vi "AlliGator Save Simulation Outputs to ASCII.vi"(8 "Error In":errorcluster, 9 "Fit Settings":T11 {"Decay Fit Options"."Confidence Level" min=0.0 max=100.0; "Decay Fit Options"."Offset Resolution" min=0.0; "Decay Fit Options"."Period" min=0.0; "Decay Fit Options"."Min Decay Percentile" min=0.0 max=1.0; "Decay Fit Options"."Max Decay Percentile" min=0.0 max=100.0; "Fit Parameter Constraints"."Max Value" format="%#.3g"; "Fit Parameter Constraints"."Min Value" format="%#.3g"}, 10 "Simulation Parameters Array":T12[](array[typedef]), 11 "Fit Results":cluster{"Fit Results":T15[]}[](array[cluster])) -> (0 "Error Out":errorcluster, 1 "Message":string)   [LabVIEW 2021, in "AlliGator Fit Method Benchmark.lvlib"]
doc: "Saves simulation results."
uses:
  AlliGator Fit Method Benchmark.lvlib
  Fits/IRF(X)PSED/IRF(X)PSED Fit Results.ctl
  AlliGator Simulation Parameters.ctl
  AlliGator Decay Simulation Parameters.ctl
  AlliGator Fit Simulation Parameters.ctl
  Fits/Decay Convolution/Decay Model.ctl
  Fits/Residual Type.ctl
  Fits/Non-linear Fitting Method v2.ctl
  Fits/Fit Calculation Method.ctl
  Fits/Non-linear Fitting Algorithm.ctl
  Decay Analysis/Decay Fit/AlliGator Decay Fit Parameter Constraints 2.ctl
  Fits/IRF(X)PSED/Decay Fit Parameters In List.ctl
  Fits/IRF(X)PSED/MLE Baseline Offset Type.ctl
  Files/Files.lvlib
  Strings/Strings.lvlib
  Fits/Fits.lvlib
  Decay Analysis/Decay Fit/AlliGator Decay Fit.lvlib
  Fits/IRF(X)PSED/Fit Weights Type v2.ctl
  Fits/IRF(X)PSED/Decay Fit Options v4.ctl
panel:
  in  "file (use dialog)":path
  # "see the AlliGator License on the block diagram (Ctrl+E or Window:Show Block Diagram)"
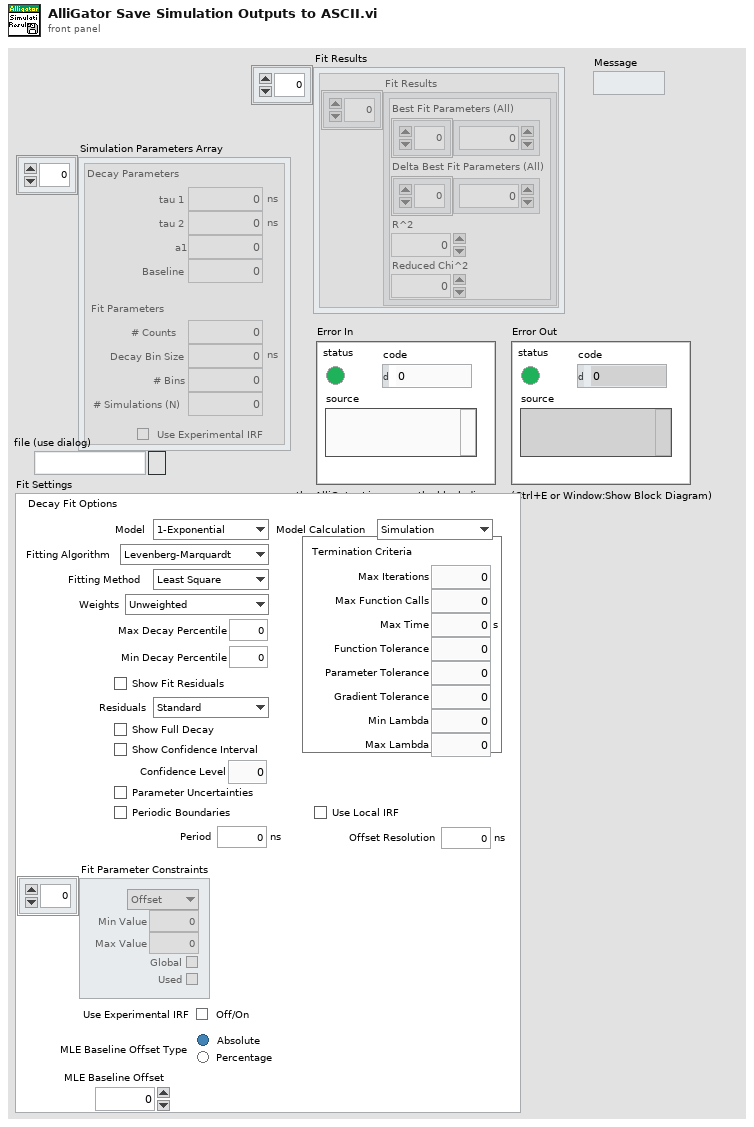
[diagram p1: front panel]
types:
  T1 = typedef "Fits.lvlib/Decay Fit Options v4.ctl" = cluster{"Show Fit Residuals":bool, "Fit Model":T2, "Residual Type":T3, "Max Decay Percentile":dbl, "Min Decay Percentile":dbl, "Show Full Decay":bool, "Weights":T4, "Fitting Method":T5, "Compute Parameter Uncertainties":bool, "Periodic Boundaries":bool, "Model Calculation":T6, "Period":dbl[unit], "Termination Criteria":cluster{"Max Iterations":i32, "Max Function Calls":i32, "Max Time":dbl[unit], "Function Tolerance":dbl, "Parameter Tolerance":dbl, "Gradient Tolerance":dbl, "Min Lambda":dbl, "Max Lambda":dbl, "Initial Tick Count":u32}, "Offset Resolution":dbl[unit], "Use Local IRF":bool, "Fitting Algorithm":T7, "Show Confidence Interval ":bool, "Confidence Level":dbl}
  T2 = typedef "Fits.lvlib/Decay Model.ctl" = enum16{"1-Exponential", "2-Exponentials"}
  T3 = typedef "Fits.lvlib/Residual Type.ctl" = enum16{"Standard", "Normalized", "Reduced"}
  T4 = typedef "Fits.lvlib/Fit Weights Type v2.ctl" = enum16{"Unweighted", "1/Variance (Neyman)", "1/Variance (Pearson)", "Best of All"}
  T5 = typedef "Fits.lvlib/Non-linear Fitting Method v2.ctl" = enum16{"Least Square", "Least Absolute Residual", "Bisquare", "MLE", "-", "Best of All"}
  T6 = typedef "Fits.lvlib/Fit Calculation Method.ctl" = enum16{"Simulation", "Convolution", "Integration"}
  T7 = typedef "Fits.lvlib/Non-linear Fitting Algorithm.ctl" = enum16{"Levenberg-Marquardt", "Trust-Region Dogleg"}
  T8 = typedef "AlliGator Decay Fit.lvlib/AlliGator Decay Fit Parameter Constraints 2.ctl" = cluster{"Fit Parameter":T9, "Min Value":dbl, "Max Value":dbl, "Global":bool, "Used":bool}
  T9 = typedef "Fits.lvlib/Decay Fit Parameters In List.ctl" = enum16{"Offset", "Baseline", "A_1", "tau_1", "A_2", "tau_2"}
  T10 = typedef "Fits.lvlib/MLE Baseline Offset Type.ctl" = enum32{"Absolute", "Percentage"}
  T11 = cluster{"Decay Fit Options":T1, "Fit Parameter Constraints":T8[], "Use Experimental IRF":bool, "MLE Baseline Offset Type":T10, "MLE Baseline Offset":dbl}
  T12 = typedef "AlliGator Fit Method Benchmark.lvlib/AlliGator Simulation Parameters.ctl" = cluster{"Decay Simulation Parameters":T13, "Fit Simulation Parameters":T14, "Use Experimental IRF":bool}
  T13 = typedef "AlliGator Fit Method Benchmark.lvlib/AlliGator Decay Simulation Parameters.ctl" = cluster{"tau 1":dbl[unit], "tau 2":dbl[unit], "a1":dbl, "Baseline":dbl}
  T14 = typedef "AlliGator Fit Method Benchmark.lvlib/AlliGator Fit Simulation Parameters.ctl" = cluster{"# Counts":i32, "# Simulations (N)":i32, "Decay Bin Size":dbl[unit], "# Bins":i32}
  T15 = typedef "Fits.lvlib/IRF(X)PSED Fit Results.ctl" = cluster{"Best Fit Parameters (All)":dbl[], "Delta Best Fit Parameters (All)":dbl[], "R^2":dbl, "Reduced Chi^2":dbl}
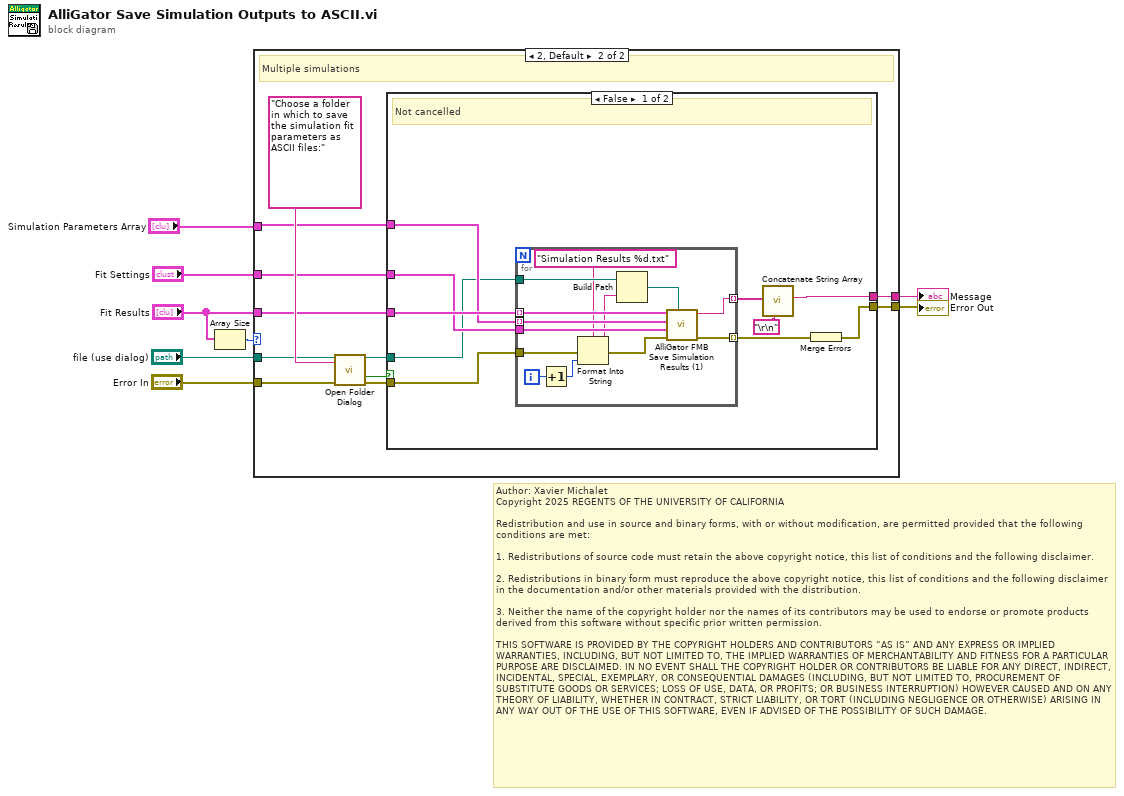
[diagram p0: block diagram]
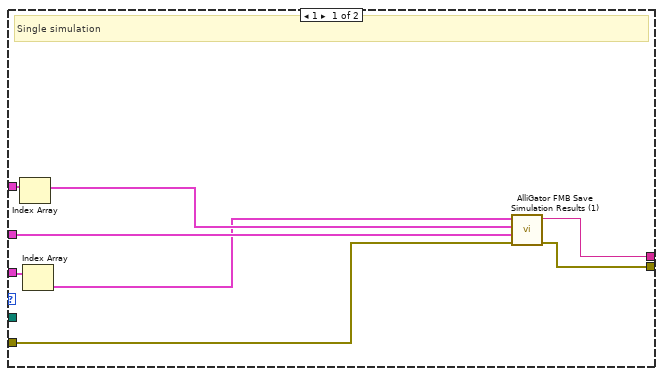
[diagram p2: hidden frame]
diagram:
  # "Author: Xavier Michalet\nCopyright 2025 REGENTS OF THE UNIVERSITY OF CALIFORNIA\n\nRedistribution and use in source and binary forms, with or without modification, are permitted provided that the following conditions are met:\n\n1. Redistributions of source code must retain the above copyright notice, this list of conditions and the following disclaimer.\n\n2. Redistributions in binary form must reproduce the above copyright notice, this list of conditions and the following disclaimer in the documentation and/or other materials provided with the distribution.\n\n3. Neither the name of the copyright holder nor the names of its contributors may be used to endorse or promote products derived from this software without specific prior written permission.\n\nTHIS SOFTWARE IS PROVIDED BY THE COPYRIGHT HOLDERS AND CONTRIBUTORS “AS IS” AND ANY EXPRESS OR IMPLIED WARRANTIES, INCLUDING, BUT NOT LIMITED TO, THE IMPLIED WARRANTIES OF MERCHANTABILITY AND FITNESS FOR A PARTICULAR PURPOSE ARE DISCLAIMED. IN NO EVENT SHALL THE COPYRIGHT HOLDER OR CONTRIBUTORS BE LIABLE FOR ANY DIRECT, INDIRECT, INCIDENTAL, SPECIAL, EXEMPLARY, OR CONSEQUENTIAL DAMAGES (INCLUDING, BUT NOT LIMITED TO, PROCUREMENT OF SUBSTITUTE GOODS OR SERVICES; LOSS OF USE, DATA, OR PROFITS; OR BUSINESS INTERRUPTION) HOWEVER CAUSED AND ON ANY THEORY OF LIABILITY, WHETHER IN CONTRACT, STRICT LIABILITY, OR TORT (INCLUDING NEGLIGENCE OR OTHERWISE) ARISING IN ANY WAY OUT OF THE USE OF THIS SOFTWARE, EVEN IF ADVISED OF THE POSSIBILITY OF SUCH DAMAGE."
  n1 = Array Size(array="Fit Results") -> (size(s)=w4:i32)
  n2 = case shown="2, Default" w4 {
    tunnel: "Error In" -> [w16 w26]
    tunnel: [w15 w17] -> w7
    tunnel: [w14 w19] -> w6
    tunnel: "Fit Results" -> [w10 w24]
    tunnel: "Simulation Parameters Array" -> [w12 w23]
    tunnel: "Fit Settings" -> [w13 w22]
    tunnel: "file (use dialog)" -> [_ w18]
    frame 1 {
      # "Single simulation"
      n3 = Index Array(array=w12) -> (element=w11:T12)  [unwired: 1 in]
      n4 = Index Array(array=w10) -> (element=w9:cluster{"Fit Results":T15[]})  [unwired: 1 in]
      n5 = call "AlliGator FMB Save Simulation Results (1).vi"("error in (no error)"=w16, "Fit Settings"=w13, "Simulation Parameters"=w11, "Fit Results"=w9) -> ("error out"=w15:errorcluster, "Message"=w14:string)  [unwired: 6 in]
    }
    frame 2, Default {
      # "Multiple simulations"
      n6 = call "Open Folder Dialog.vi"("start path"=w18, "prompt"="Choose a folder in which to save the simulation fit parameters as ASCII files:" ("prompt (Choose or enter file path)"), "error in"=w26) -> ("selected path"=w20:path, "cancelled"=w25:bool, "error out"=w21:errorcluster)  [unwired: 9 in, 1 out]
      n7 = case shown="False" w25 {
        tunnel: w24 -> [w37 _]
        tunnel: w23 -> [w36 _]
        tunnel: w22 -> [w35 _]
        tunnel: w21 -> [w34 w51]
        tunnel: w20 -> [w30 _]
        tunnel: [w32 _] -> w19
        tunnel: [w28 w51] -> w17
        frame False {
          # "Not cancelled"
          n8 = for {
            tunnel: w37 -> [w50] mode=indexing
            tunnel: w36 -> [w49] mode=indexing
            tunnel: w35 -> [w48]
            tunnel: w34 -> [w43]
            tunnel: [w47] -> w29 mode=indexing
            tunnel: [w46] -> w33 mode=indexing
            tunnel: w30 -> [w45]
            i -> [w42]
            n9 = Increment(x=w42) -> (x+1=w41:i32)
            n10 = Format Into String(format string="Simulation Results %d.txt", error in=w43, w41) -> (resulting string=w39:string, error out=w44:errorcluster)  [unwired: 1 in]
            n11 = Build Path(base path=w45, name or relative path=w39) -> (appended path=w38:path)
            n12 = call "AlliGator FMB Save Simulation Results (1).vi"("File Path (Dialog if empty)"=w38, "error in (no error)"=w44, "Fit Settings"=w48, "Simulation Parameters"=w49, "Fit Results"=w50) -> ("error out"=w47:errorcluster, "Message"=w46:string)  [unwired: 5 in]
          }
          n13 = call "Concatenate String Array.vi"("Separator (TAB)"="\r\n", "String Array"=w33) -> ("Formatted String"=w32:string)  [unwired: 9 in]
          n14 = Merge Errors(w29) -> (w28:errorcluster)
        }
        frame True {
          # "Cancelled"
        }
      }
    }
  }
  "Error Out" <- w7
  "Message" <- w6
